vi "split u8 into lower middle and upper bits.vi"(11 "Numeric":u8=3) -> (1 "upper 2 bits as number for red":u8, 2 "middle 2 bits as number for green":u8, 3 "lower 3 bits as number for blue":u8)   [LabVIEW 2020]
doc: "Splits the u8 representing an ascii character into 7 bits (2 bits for red, 2 bits for green, and 3 bits for blue) to be encoded into the LSBs of a pixel expressed in 24 bits (1 byte r, 1 byte g, 1 byte b)."
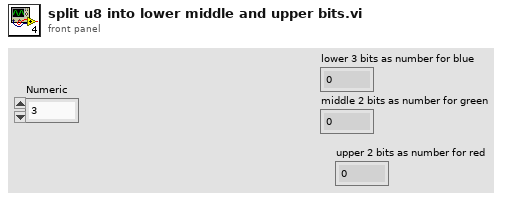
[diagram p1: front panel]
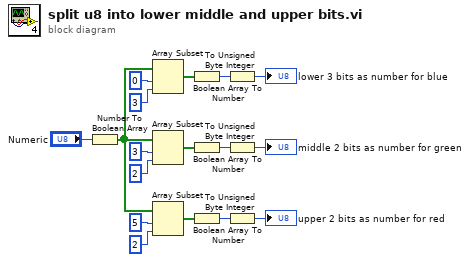
[diagram p0: block diagram]
diagram:
  n1 = Number To Boolean Array(number="Numeric") -> (Boolean array=w10:bool[])
  n2 = Array Subset(array=w10, index=0, length=3) -> (w9:bool[])
  n3 = Array Subset(array=w10, index=3, length=2) -> (w4:bool[])
  n4 = Array Subset(array=w10, index=5, length=2) -> (w1:bool[])
  n5 = Boolean Array To Number(Boolean array=w9) -> (number=w8:u32)
  n6 = Boolean Array To Number(Boolean array=w4) -> (number=w6:u32)
  n7 = Boolean Array To Number(Boolean array=w1) -> (number=w2:u32)
  n8 = To Unsigned Byte Integer(number=w8) -> (unsigned 8bit integer=→"lower 3 bits as number for blue":u8)
  n9 = To Unsigned Byte Integer(number=w6) -> (unsigned 8bit integer=→"middle 2 bits as number for green":u8)
  n10 = To Unsigned Byte Integer(number=w2) -> (unsigned 8bit integer=→"upper 2 bits as number for red":u8)
